vi "Find free COM ports.vi"() -> (3 "Free COM ports":string[](array[string]))   [LabVIEW 2021, in "F-70 driver.lvlib"]
doc: "Returns an array of free COM ports."
uses:
  F-70 driver.lvlib
  <vilib>/Instr/_visa.llb/VISA Find Search Mode.ctl
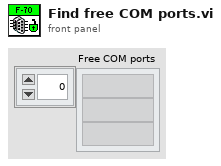
[diagram p1: front panel]
types:
  T1 = typedef "VISA Find Search Mode.ctl" = u32
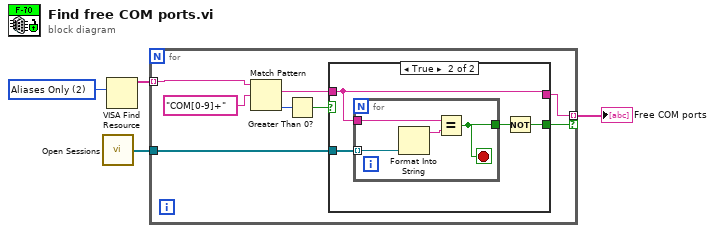
[diagram p0: block diagram]
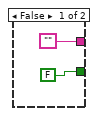
[diagram p2: hidden frame]
diagram:
  w2 = T1 2 items=["Canonical Names Only"=0, "Aliases Only"=2, "Include Matching Aliases"=3, "Include All Aliases"=4] ("Search Mode")
  n1 = call <vilib>:"Open Sessions.vi"() -> ("Array of Refnums"=w3:refnum<visa-resource-name>[])  [unwired: 2 in]
  n2 = VISA Find Resource(10:w2) -> (3:w1:string[])  [unwired: 2 in, 2 out]
  n3 = for {
    tunnel: w1 -> [w11] mode=indexing
    tunnel: w3 -> [w7]
    tunnel: [w6] -> w4 mode=indexing if=w5
    n4 = Match Pattern(string=w11, regular expression="COM[0-9]+") -> (match substring=w8:string, offset past match=w10:i32)  [unwired: 1 in, 2 out]
    n5 = Greater Than 0?(x=w10) -> (x > 0?=w9:bool)
    n6 = case shown="True" w9 {
      tunnel: w8 -> [_ w15]
      tunnel: w7 -> [_ w18]
      tunnel: [FALSE w16] -> w5
      tunnel: ["" ("String") w15] -> w6
      frame False {
      }
      frame True {
        n7 = for {
          tunnel: w18 -> [w22] mode=indexing
          tunnel: w15 -> [w20]
          tunnel: [w21] -> w17
          stop <- w21 stop-if-true
          n8 = Format Into String(w22) -> (resulting string=w19:string)  [unwired: 3 in, 1 out]
          n9 = Equal?(x=w20, y=w19) -> (x = y?=w21:bool)
        }
        n10 = Not(x=w17) -> (.not. x?=w16:bool)
      }
    }
  }
  "Free COM ports" <- w4
